vi "5492_CollectButtons.vi"() -> ()   [LabVIEW 2017]
panel:
  in  "Heelies":bool
  in  "The Claw":bool
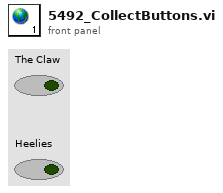
[diagram p1: front panel]
diagram:
